vi "Open Motors.vi"   [LabVIEW 2018]
uses:
  <vilib>/Rock Robotics/WPI/RobotDrive/WPI_RobotDriveOpen4MotorWithExistingMotors.vi
types:
  T1 = typedef "WPI_MotorControlDeviceRef.ctl" = cluster{"DeviceStatus":errorcluster, "Type":T2, "PWM":cluster{"PWM Channel":T3, "DeadBand":T4}, "CAN":cluster{"Device Number":u8, "SetOutput VI Ref":variant, "GetOutput VI Ref":variant, "Enable VI Ref":variant, "Disable VI Ref":variant, "Data":variant}, "Invert":bool, "DIO PWM":cluster{"PWM \"Enable\" Channel":T3, "DIOChannel":T5, "PWM Rate":dbl}}
  T2 = typedef "WPI_MotorControlType.ctl" = enum16{"PWM", "CAN", "DIO PWM"}
  T3 = typedef "FPGA_DIOPWMChannel.ctl" = enum8{"PWM 0", "PWM 1", "PWM 2", "PWM 3", "PWM 4", "PWM 5", "PWM 6", "PWM 7", "PWM 8", "PWM 9", "PWM MXP 0", "PWM MXP 1", "PWM MXP 2", "PWM MXP 3", "PWM MXP 4", "PWM MXP 5", "PWM MXP 6", "PWM MXP 7", "PWM MXP 8", "PWM MXP 9", "Invalid"}
  T4 = typedef "WPI_PWMDeadband.ctl" = cluster{"Name":string, "maxPositivePwm":i32, "minPositivePwm":i32, "centerPwm":i32, "maxNegativePwm":i32, "minNegativePwm":i32, "angularRange":u16}
  T5 = typedef "FPGA_DIOChannel.ctl" = enum8{"DIO 0", "DIO 1", "DIO 2", "DIO 3", "DIO 4", "DIO 5", "DIO 6", "DIO 7", "DIO 8", "DIO 9", "DIO MXP 0", "DIO MXP 1", "DIO MXP 2", "DIO MXP 3", "DIO MXP 4", "DIO MXP 5", "DIO MXP 6", "DIO MXP 7", "DIO MXP 8", "DIO MXP 9", "DIO MXP 10", "DIO MXP 11", "DIO MXP 12", "DIO MXP 13", "DIO MXP 14", "DIO MXP 15", "SPI Port CS1", "SPI Port CS2", "SPI Port CS3", "SPI Port MISO", "SPI Port MOSI", "Invalid"}
  T6 = typedef "WPI_RobotDriveDevRef.ctl" = cluster{"DevStatus":errorcluster, "Motors[]":T1[], "Square Inputs":bool, "Max Output":dbl}
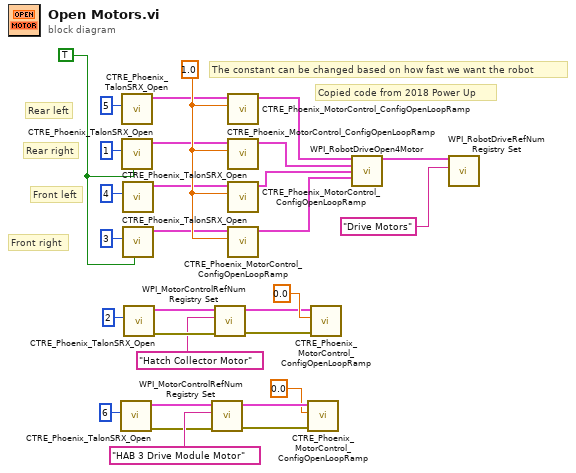
[diagram p0: block diagram]
diagram:
  w8 = TRUE
  w17 = 1.0
  # "Front right"
  # "Front left"
  # "Rear right"
  # "Rear left"
  # "Copied code from 2018 Power Up"
  # "The constant can be changed based on how fast we want the robot"
  n1 = call <vilib>:"CTRE_Phoenix_TalonSRX_Open.vi"("Device Number"=u8 6) -> ("error out"=w3:errorcluster, "CAN Talon SRX Ref"=w6:T1)  [unwired: 9 in]
  n2 = call <vilib>:"CTRE_Phoenix_TalonSRX_Open.vi"("Device Number"=u8 5) -> ("CAN Talon SRX Ref"=w10:T1)  [unwired: 9 in, 1 out]
  n3 = call <vilib>:"CTRE_Phoenix_TalonSRX_Open.vi"("Invert"=w8, "Device Number"=u8 1) -> ("CAN Talon SRX Ref"=w11:T1)  [unwired: 8 in, 1 out]
  n4 = call <vilib>:"CTRE_Phoenix_TalonSRX_Open.vi"("Device Number"=u8 4) -> ("CAN Talon SRX Ref"=w15:T1)  [unwired: 9 in, 1 out]
  n5 = call <vilib>:"CTRE_Phoenix_TalonSRX_Open.vi"("Invert"=w8, "Device Number"=u8 3) -> ("CAN Talon SRX Ref"=w14:T1)  [unwired: 8 in, 1 out]
  n6 = call <vilib>:"CTRE_Phoenix_TalonSRX_Open.vi"("Device Number"=u8 2) -> ("error out"=w28:errorcluster, "CAN Talon SRX Ref"=w25:T1)  [unwired: 9 in]
  n7 = call <vilib>:"WPI_MotorControlRefNum Registry Set.vi"("error in (no error)"=w3, "refnum name"="HAB 3 Drive Module Motor", "MotorControlDevRef"=w6) -> ("error out"=w2:errorcluster, "MotorControlDevRef"=w4:T1)  [unwired: 7 in]
  n8 = call <vilib>:"WPI_MotorControlRefNum Registry Set.vi"("error in (no error)"=w28, "refnum name"="Hatch Collector Motor", "MotorControlDevRef"=w25) -> ("error out"=w29:errorcluster, "MotorControlDevRef"=w27:T1)  [unwired: 7 in]
  n9 = call <vilib>:"CTRE_Phoenix_MotorControl_ConfigOpenLoopRamp.vi"("secondsFromNeutralToFull"=w17, "PhoenixMotorControlDevRef"=w10) -> ("PhoenixMotorControlDevRef"=w18:T1)  [unwired: 8 in, 1 out]
  n10 = call <vilib>:"CTRE_Phoenix_MotorControl_ConfigOpenLoopRamp.vi"("secondsFromNeutralToFull"=w17, "PhoenixMotorControlDevRef"=w11) -> ("PhoenixMotorControlDevRef"=w19:T1)  [unwired: 8 in, 1 out]
  n11 = call <vilib>:"CTRE_Phoenix_MotorControl_ConfigOpenLoopRamp.vi"("secondsFromNeutralToFull"=w17, "PhoenixMotorControlDevRef"=w15) -> ("PhoenixMotorControlDevRef"=w20:T1)  [unwired: 8 in, 1 out]
  n12 = call <vilib>:"CTRE_Phoenix_MotorControl_ConfigOpenLoopRamp.vi"("secondsFromNeutralToFull"=w17, "PhoenixMotorControlDevRef"=w14) -> ("PhoenixMotorControlDevRef"=w21:T1)  [unwired: 8 in, 1 out]
  n13 = call <vilib>:"CTRE_Phoenix_MotorControl_ConfigOpenLoopRamp.vi"("error in (no error)"=w2, "secondsFromNeutralToFull"=0.0, "PhoenixMotorControlDevRef"=w4) -> ()  [unwired: 7 in, 2 out]
  n14 = call <vilib>:"CTRE_Phoenix_MotorControl_ConfigOpenLoopRamp.vi"("error in (no error)"=w29, "secondsFromNeutralToFull"=0.0, "PhoenixMotorControlDevRef"=w27) -> ()  [unwired: 7 in, 2 out]
  n15 = call-poly <vilib>:"WPI_RobotDriveOpen4Motor.vi"("Rear Left Motor Dev Ref"=w18, "Rear Right Motor Dev Ref"=w19, "Front Left Motor Dev Ref"=w20, "Front Right Motor Dev Ref"=w21) -> ("RobotDriveDevRef"=w22:T6)  [unwired: 10 in, 1 out]
  n16 = call <vilib>:"WPI_RobotDriveRefNum Registry Set.vi"("refnum name"="Drive Motors", "RobotDriveDevRef"=w22) -> ()  [unwired: 8 in, 2 out]
